vi "BT Tx Test Get Default USL.vi"(8 "error in (no error)":errorcluster, 11 "Template Tx Test in":refnum<class "niDTS BT Tx Test.lvclass">) -> (0 "error out":errorcluster, 2 "Default USL":T1 {"OBW Resutls"."Stop Frequency (Hz)" format="%#_4p"; "OBW Resutls"."Start Frequency (Hz)" format="%#_4p"}, 3 "Template Tx Test out":refnum<class "niDTS BT Tx Test.lvclass">)   [LabVIEW 2015, in "niDTS BT.lvlib" / "niDTS BT Tx Test.lvclass"]
uses:
  niDTS BT Tx Test.lvclass
  Includes/niDTS BT Tx Test INC Results.ctl
  Includes/niDTS BT Tx Test INC IBE Results.ctl
  Includes/niDTS BT Tx Test INC OBW Results.ctl
  Includes/niDTS BT Tx Test INC TXP Results.ctl
  Includes/niDTS BT Tx Test INC DEVM Results.ctl
  Includes/niDTS BT Tx Test INC CF Stability Results.ctl
  Includes/niDTS BT Tx Test INC CFO Resutls.ctl
  Includes/niDTS BT Tx Test INC Character Results.ctl
  niDTS BT Tx Test.lvclass/niDTS BT Tx Test.ctl
  Includes/niDTS BT Tx Test INC Default Limits.vi
  niDTS BT.lvlib
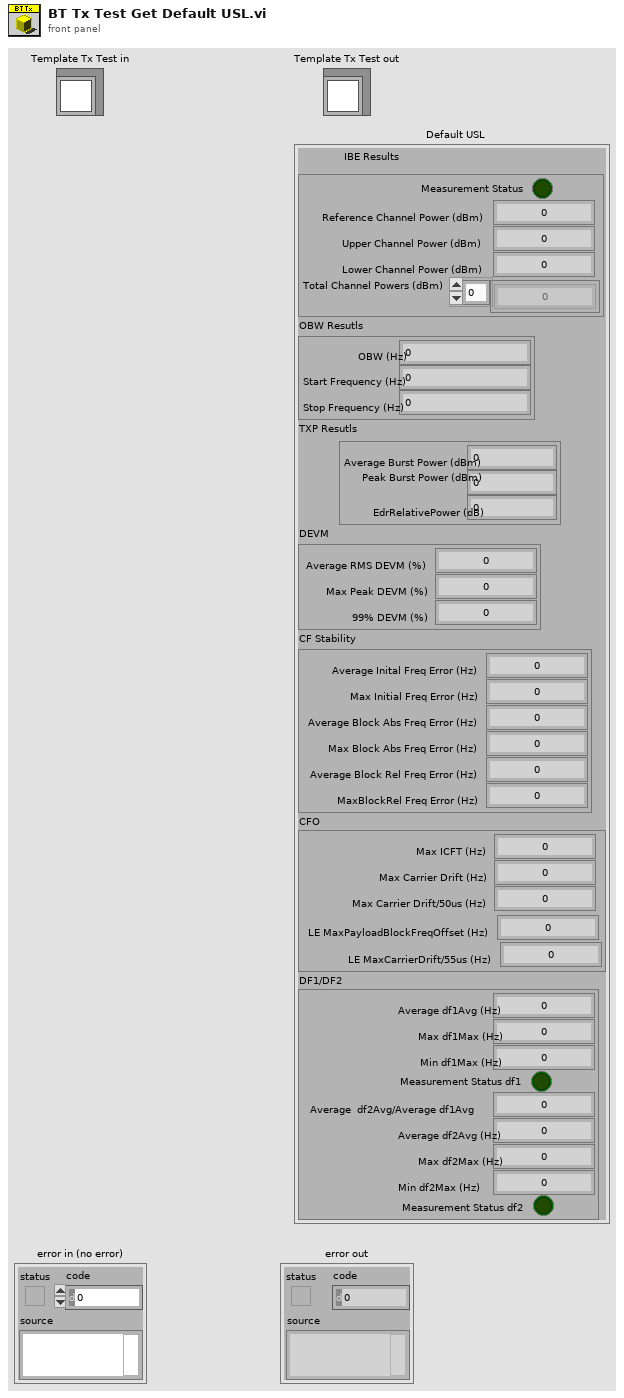
[diagram p1: front panel]
types:
  T1 = typedef "niDTS BT.lvlib/niDTS BT Tx Test INC Results.ctl" = cluster{"IBE Results":T2, "OBW Resutls":T3, "TXP Resutls":T4, "DEVM":T5, "CF Stability":T6, "CFO":T7, "DF1/DF2":T8}
  T2 = typedef "niDTS BT.lvlib/niDTS BT Tx Test INC IBE Results.ctl" = cluster{"Measurement Status":bool, "Reference Channel Power (dBm)":dbl, "Upper Channel Power (dBm)":dbl, "Lower Channel Power (dBm)":dbl, "Total Channel Powers (dBm)":dbl[]}
  T3 = typedef "niDTS BT.lvlib/niDTS BT Tx Test INC OBW Results.ctl" = cluster{"OBW (Hz)":dbl, "Start Frequency (Hz)":dbl, "Stop Frequency (Hz)":dbl}
  T4 = typedef "niDTS BT.lvlib/niDTS BT Tx Test INC TXP Results.ctl" = cluster{"Average Burst Power (dBm)":dbl, "Peak Burst Power (dBm)":dbl, "EdrRelativePower (dB)":dbl}
  T5 = typedef "niDTS BT.lvlib/niDTS BT Tx Test INC DEVM Results.ctl" = cluster{"Average RMS DEVM (%)":dbl, "Max Peak DEVM (%)":dbl, "99% DEVM (%)":dbl}
  T6 = typedef "niDTS BT.lvlib/niDTS BT Tx Test INC CF Stability Results.ctl" = cluster{"Average Inital Freq Error (Hz)":dbl, "Max Initial Freq Error (Hz)":dbl, "Average Block Abs Freq Error (Hz)":dbl, "Max Block Abs Freq Error (Hz)":dbl, "Average Block Rel Freq Error (Hz)":dbl, "MaxBlockRel Freq Error (Hz)":dbl}
  T7 = typedef "niDTS BT.lvlib/niDTS BT Tx Test INC CFO Resutls.ctl" = cluster{"Max ICFT (Hz)":dbl, "Max Carrier Drift (Hz)":dbl, "Max Carrier Drift/50us (Hz)":dbl, "LE MaxPayloadBlockFreqOffset (Hz)":dbl, "LE MaxCarrierDrift/55us (Hz)":dbl}
  T8 = typedef "niDTS BT.lvlib/niDTS BT Tx Test INC Character Results.ctl" = cluster{"Average df1Avg (Hz)":dbl, "Max df1Max (Hz)":dbl, "Min df1Max (Hz)":dbl, "Measurement Status df1":bool, "Average  df2Avg/Average df1Avg":dbl, "Average df2Avg (Hz)":dbl, "Max df2Max (Hz)":dbl, "Min df2Max (Hz)":dbl, "Measurement Status df2":bool}
  T9 = typedef "niDTS BT.lvlib/niDTS BT INC Packet Type.ctl" = enum16{"NULL", "POLL", "FHS", "DM1", "DH1", "HV1", "HV2", "HV3", "EV3", "DV", "AUX1", "DM3", "DH3", "EV4", "EV5", "DM5", "DH5", "LE-TP"}
  T10 = typedef "niDTS BT.lvlib/niDTS BT INC Standard.ctl" = enum16{"BDR", "EDR", "LE-TP"}
  T11 = typedef "niDTS BT.lvlib/niDTS BT Tx Test INC BD Payload Data.ctl" = enum16{"0", "1", "01", "00001111", "PN9", "AUTO"}
  T12 = typedef "niDTS BT.lvlib/niDTS BT Tx Test INC Modulation Characteristics.ctl" = enum16{"DF1", "DF2", "BOTH"}
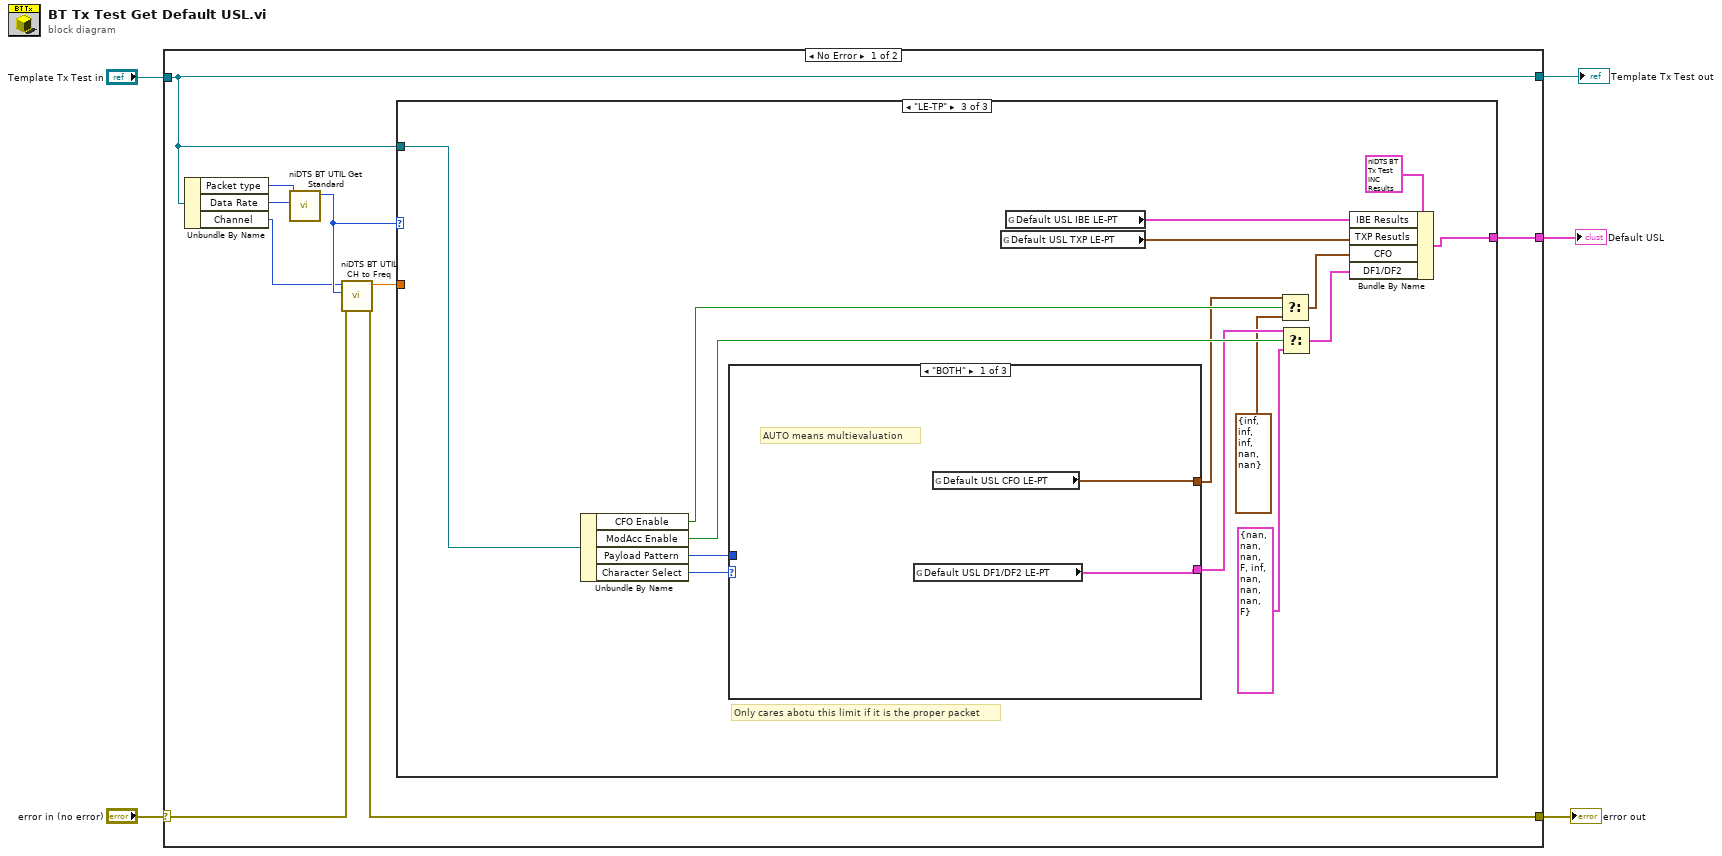
[diagram p0: block diagram]
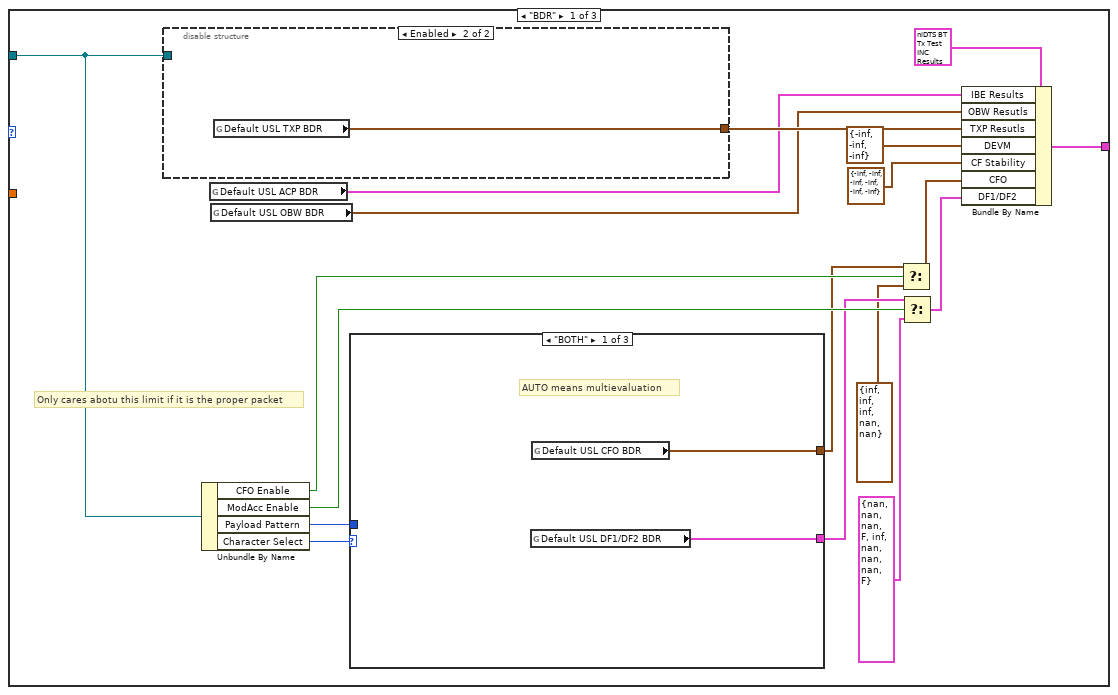
[diagram p2: hidden frame]
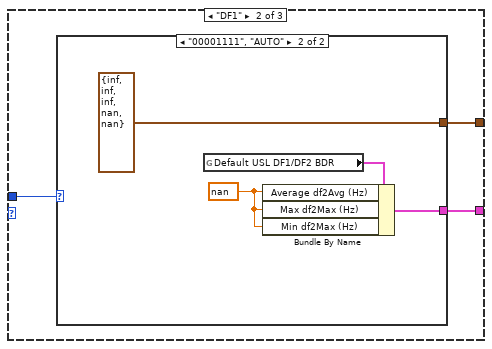
[diagram p3: hidden frame]
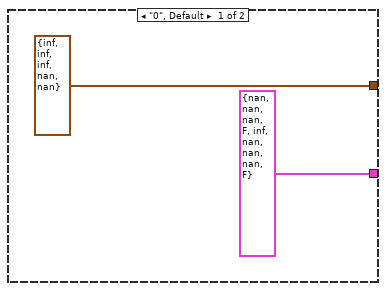
[diagram p4: hidden frame]
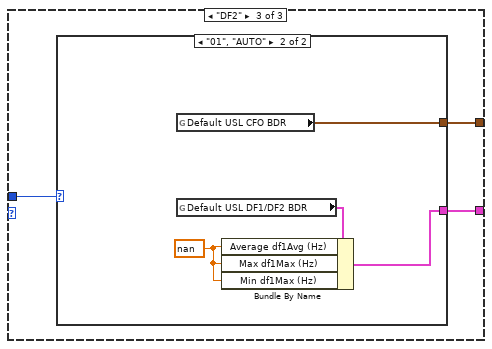
[diagram p5: hidden frame]
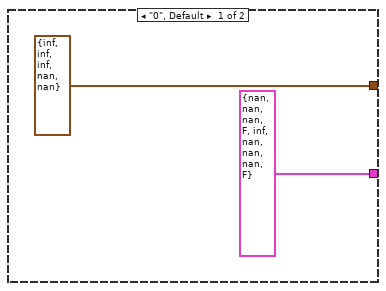
[diagram p6: hidden frame]
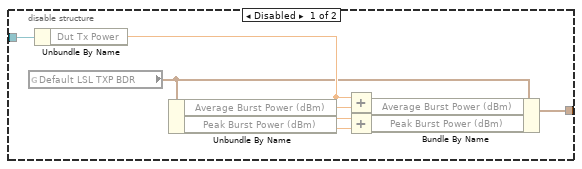
[diagram p7: hidden frame]
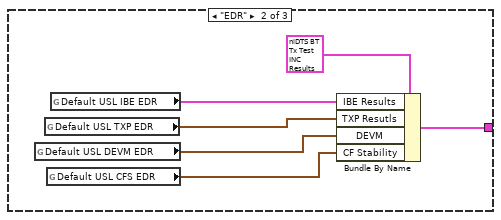
[diagram p8: hidden frame]
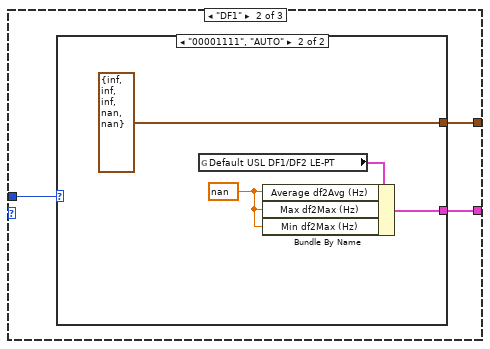
[diagram p9: hidden frame]
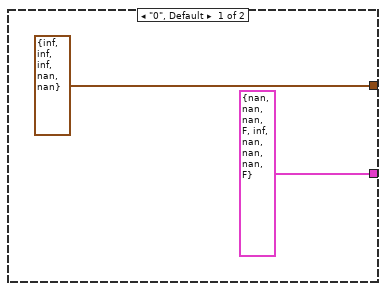
[diagram p10: hidden frame]
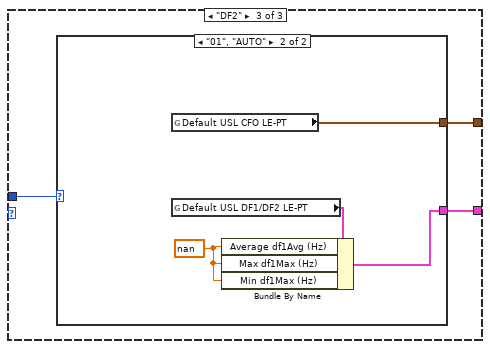
[diagram p11: hidden frame]
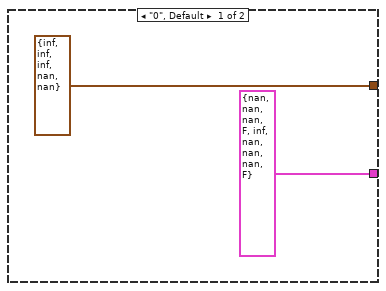
[diagram p12: hidden frame]
diagram:
  n1 = case shown="No Error" "error in (no error)" {
    selector: "error in (no error)" -> [w8 w104]
    tunnel: [w7 w104] -> w1
    tunnel: [w13 w103] -> w3
    tunnel: "Template Tx Test in" -> [w13 w103]
    tunnel: [w14 _] -> w2
    frame No Error {
      n2 = Unbundle By Name(w13) -> ("Packet type"=w11:T9, "Data Rate"=w12:i32, "Channel"=w9:i32)
      n3 = call "niDTS BT UTIL Get Standard.vi"("Data Rate"=w12, "Packet type"=w11) -> ("BT Standard"=w10:T10)  [unwired: 9 in]
      n4 = call "niDTS BT UTIL CH to Freq.vi"("error in (no error)"=w8, "BT Standard"=w10, "Channel"=w9) -> ("error out"=w7:errorcluster, "Frequency"=w6:dbl)  [unwired: 7 in]
      n5 = case shown="\"LE-TP\"" w10 {
        tunnel: [w30 w62 w80] -> w14
        tunnel: w13 -> [w25 _ w71]
        tunnel: w6 -> [_ _ _]
        frame "BDR" {
          # "Only cares abotu this limit if it is the proper packet"
          n6 = disable-structure shown="Enabled" {
            disable-tunnel: w25 -> [w60 _]
            disable-tunnel: [w54 w61] -> w31
            frame Disabled {
              n7 = global read "niDTS BT Tx Test INC Default Limits.vi" "Default LSL TXP BDR"() -> (w53:T4)
              n8 = Unbundle By Name(w60) -> ("Dut Tx Power"=w58:dbl)
              n9 = Unbundle By Name(w53) -> ("Average Burst Power (dBm)"=w59:dbl, "Peak Burst Power (dBm)"=w57:dbl)
              n10 = Add(x=w58, y=w59) -> (x+y=w56:dbl)
              n11 = Add(x=w58, y=w57) -> (x+y=w55:dbl)
              n12 = Bundle By Name(cluster=w53, "Average Burst Power (dBm)"=w56, "Peak Burst Power (dBm)"=w55) -> (w54:T4)
            }
            frame Enabled {
              n13 = global read "niDTS BT Tx Test INC Default Limits.vi" "Default USL TXP BDR"() -> (w61:T4)
            }
          }
          n14 = Unbundle By Name(w25) -> ("CFO Enable"=w23:bool, "ModAcc Enable"=w22:bool, "Payload Pattern"=w24:T11, "Character Select"=w15:T12)
          n15 = global read "niDTS BT Tx Test INC Default Limits.vi" "Default USL ACP BDR"() -> (w29:T2)
          n16 = global read "niDTS BT Tx Test INC Default Limits.vi" "Default USL OBW BDR"() -> (w26:T3)
          n17 = case shown="\"BOTH\"" w15 {
            tunnel: [w33 w37 w46] -> w19
            tunnel: w24 -> [_ w36 w45]
            tunnel: [w34 w35 w44] -> w21
            frame "BOTH" {
              # "AUTO means multievaluation"
              n18 = global read "niDTS BT Tx Test INC Default Limits.vi" "Default USL DF1/DF2 BDR"() -> (w33:T8)
              n19 = global read "niDTS BT Tx Test INC Default Limits.vi" "Default USL CFO BDR"() -> (w34:T7)
            }
            frame "DF1" {
              n20 = case shown="\"00001111\", \"AUTO\"" w36 {
                tunnel: [T8 {"Average df1Avg (Hz)"=nan, "Max df1Max (Hz)"=nan, "Min df1Max (Hz)"=nan, "Measurement Status df1"=FALSE, "Average  df2Avg/Average df1Avg"=inf, "Average df2Avg (Hz)"=nan, "Max df2Max (Hz)"=nan, "Min df2Max (Hz)"=nan, "Measurement Status df2"=FALSE} ("Default USL DF1/DF2 BDR") w41] -> w37
                tunnel: [T7 {"Max ICFT (Hz)"=inf, "Max Carrier Drift (Hz)"=inf, "Max Carrier Drift/50us (Hz)"=inf, "LE MaxPayloadBlockFreqOffset (Hz)"=nan, "LE MaxCarrierDrift/55us (Hz)"=nan} ("f") T7 {"Max ICFT (Hz)"=inf, "Max Carrier Drift (Hz)"=inf, "Max Carrier Drift/50us (Hz)"=inf, "LE MaxPayloadBlockFreqOffset (Hz)"=nan, "LE MaxCarrierDrift/55us (Hz)"=nan} ("f")] -> w35
                frame "0", Default {
                }
                frame "00001111", "AUTO" {
                  w42 = nan ("Average df1Avg")
                  n21 = global read "niDTS BT Tx Test INC Default Limits.vi" "Default USL DF1/DF2 BDR"() -> (w43:T8)
                  n22 = Bundle By Name(cluster=w43, "Average df2Avg (Hz)"=w42, "Max df2Max (Hz)"=w42, "Min df2Max (Hz)"=w42) -> (w41:T8)
                }
              }
            }
            frame "DF2" {
              n23 = case shown="\"01\", \"AUTO\"" w45 {
                tunnel: [T8 {"Average df1Avg (Hz)"=nan, "Max df1Max (Hz)"=nan, "Min df1Max (Hz)"=nan, "Measurement Status df1"=FALSE, "Average  df2Avg/Average df1Avg"=inf, "Average df2Avg (Hz)"=nan, "Max df2Max (Hz)"=nan, "Min df2Max (Hz)"=nan, "Measurement Status df2"=FALSE} ("Default USL DF1/DF2 BDR") w50] -> w46
                tunnel: [T7 {"Max ICFT (Hz)"=inf, "Max Carrier Drift (Hz)"=inf, "Max Carrier Drift/50us (Hz)"=inf, "LE MaxPayloadBlockFreqOffset (Hz)"=nan, "LE MaxCarrierDrift/55us (Hz)"=nan} ("f") w49] -> w44
                frame "0", Default {
                }
                frame "01", "AUTO" {
                  w51 = nan ("Average df1Avg")
                  n24 = global read "niDTS BT Tx Test INC Default Limits.vi" "Default USL CFO BDR"() -> (w49:T7)
                  n25 = global read "niDTS BT Tx Test INC Default Limits.vi" "Default USL DF1/DF2 BDR"() -> (w52:T8)
                  n26 = Bundle By Name(cluster=w52, "Average df1Avg (Hz)"=w51, "Max df1Max (Hz)"=w51, "Min df1Max (Hz)"=w51) -> (w50:T8)
                }
              }
            }
          }
          n27 = Select(t=w21, s=w23, f=T7 {"Max ICFT (Hz)"=inf, "Max Carrier Drift (Hz)"=inf, "Max Carrier Drift/50us (Hz)"=inf, "LE MaxPayloadBlockFreqOffset (Hz)"=nan, "LE MaxCarrierDrift/55us (Hz)"=nan}) -> (s? t:f=w20:T7)
          n28 = Select(t=w19, s=w22, f=T8 {"Average df1Avg (Hz)"=nan, "Max df1Max (Hz)"=nan, "Min df1Max (Hz)"=nan, "Measurement Status df1"=FALSE, "Average  df2Avg/Average df1Avg"=inf, "Average df2Avg (Hz)"=nan, "Max df2Max (Hz)"=nan, "Min df2Max (Hz)"=nan, "Measurement Status df2"=FALSE} ("Default USL DF1/DF2 BDR")) -> (s? t:f=w18:T8)
          n29 = Bundle By Name(cluster=T1 {"IBE Results"={"Measurement Status"=FALSE, "Reference Channel Power (dBm)"=0.0, "Upper Channel Power (dBm)"=0.0, "Lower Channel Power (dBm)"=0.0, "Total Channel Powers (dBm)"=[]}, "OBW Resutls"={"OBW (Hz)"=0.0, "Start Frequency (Hz)"=0.0, "Stop Frequency (Hz)"=0.0}, "TXP Resutls"={"Average Burst Power (dBm)"=-35.0, "Peak Burst Power (dBm)"=-35.0, "EdrRelativePower (dB)"=0.0}, "DEVM"={"Average RMS DEVM (%)"=0.0, "Max Peak DEVM (%)"=0.0, "99% DEVM (%)"=0.0}, "CF Stability"={"Average Inital Freq Error (Hz)"=0.0, "Max Initial Freq Error (Hz)"=0.0, "Average Block Abs Freq Error (Hz)"=0.0, "Max Block Abs Freq Error (Hz)"=0.0, "Average Block Rel Freq Error (Hz)"=0.0, "MaxBlockRel Freq Error (Hz)"=0.0}, "CFO"={"Max ICFT (Hz)"=0.0, "Max Carrier Drift (Hz)"=0.0, "Max Carrier Drift/50us (Hz)"=0.0, "LE MaxPayloadBlockFreqOffset (Hz)"=0.0, "LE MaxCarrierDrift/55us (Hz)"=0.0}, "DF1/DF2"={"Average df1Avg (Hz)"=0.0, "Max df1Max (Hz)"=0.0, "Min df1Max (Hz)"=0.0, "Measurement Status df1"=FALSE, "Average  df2Avg/Average df1Avg"=0.0, "Average df2Avg (Hz)"=0.0, "Max df2Max (Hz)"=0.0, "Min df2Max (Hz)"=0.0, "Measurement Status df2"=FALSE}} ("Default USL"), "IBE Results"=w29, "OBW Resutls"=w26, "TXP Resutls"=w31, "DEVM"=T5 {"Average RMS DEVM (%)"=-inf, "Max Peak DEVM (%)"=-inf, "99% DEVM (%)"=-inf}, "CF Stability"=T6 {"Average Inital Freq Error (Hz)"=-inf, "Max Initial Freq Error (Hz)"=-inf, "Average Block Abs Freq Error (Hz)"=-inf, "Max Block Abs Freq Error (Hz)"=-inf, "Average Block Rel Freq Error (Hz)"=-inf, "MaxBlockRel Freq Error (Hz)"=-inf}, "CFO"=w20, "DF1/DF2"=w18) -> (w30:T1)
        }
        frame "EDR" {
          n30 = global read "niDTS BT Tx Test INC Default Limits.vi" "Default USL DEVM EDR"() -> (w64:T5)
          n31 = global read "niDTS BT Tx Test INC Default Limits.vi" "Default USL TXP EDR"() -> (w63:T4)
          n32 = global read "niDTS BT Tx Test INC Default Limits.vi" "Default USL CFS EDR"() -> (w65:T6)
          n33 = global read "niDTS BT Tx Test INC Default Limits.vi" "Default USL IBE EDR"() -> (w66:T2)
          n34 = Bundle By Name(cluster=T1 {"IBE Results"={"Measurement Status"=FALSE, "Reference Channel Power (dBm)"=0.0, "Upper Channel Power (dBm)"=0.0, "Lower Channel Power (dBm)"=0.0, "Total Channel Powers (dBm)"=[]}, "OBW Resutls"={"OBW (Hz)"=0.0, "Start Frequency (Hz)"=0.0, "Stop Frequency (Hz)"=0.0}, "TXP Resutls"={"Average Burst Power (dBm)"=-35.0, "Peak Burst Power (dBm)"=-35.0, "EdrRelativePower (dB)"=0.0}, "DEVM"={"Average RMS DEVM (%)"=0.0, "Max Peak DEVM (%)"=0.0, "99% DEVM (%)"=0.0}, "CF Stability"={"Average Inital Freq Error (Hz)"=0.0, "Max Initial Freq Error (Hz)"=0.0, "Average Block Abs Freq Error (Hz)"=0.0, "Max Block Abs Freq Error (Hz)"=0.0, "Average Block Rel Freq Error (Hz)"=0.0, "MaxBlockRel Freq Error (Hz)"=0.0}, "CFO"={"Max ICFT (Hz)"=0.0, "Max Carrier Drift (Hz)"=0.0, "Max Carrier Drift/50us (Hz)"=0.0, "LE MaxPayloadBlockFreqOffset (Hz)"=0.0, "LE MaxCarrierDrift/55us (Hz)"=0.0}, "DF1/DF2"={"Average df1Avg (Hz)"=0.0, "Max df1Max (Hz)"=0.0, "Min df1Max (Hz)"=0.0, "Measurement Status df1"=FALSE, "Average  df2Avg/Average df1Avg"=0.0, "Average df2Avg (Hz)"=0.0, "Max df2Max (Hz)"=0.0, "Min df2Max (Hz)"=0.0, "Measurement Status df2"=FALSE}} ("Default USL"), "IBE Results"=w66, "TXP Resutls"=w63, "DEVM"=w64, "CF Stability"=w65) -> (w62:T1)
        }
        frame "LE-TP" {
          # "Only cares abotu this limit if it is the proper packet"
          n35 = Unbundle By Name(w71) -> ("CFO Enable"=w78:bool, "ModAcc Enable"=w77:bool, "Payload Pattern"=w79:T11, "Character Select"=w72:T12)
          n36 = case shown="\"BOTH\"" w72 {
            tunnel: [w83 w87 w96] -> w75
            tunnel: w79 -> [_ w86 w95]
            tunnel: [w84 w85 w94] -> w76
            frame "BOTH" {
              # "AUTO means multievaluation"
              n37 = global read "niDTS BT Tx Test INC Default Limits.vi" "Default USL DF1/DF2 LE-PT"() -> (w83:T8)
              n38 = global read "niDTS BT Tx Test INC Default Limits.vi" "Default USL CFO LE-PT"() -> (w84:T7)
            }
            frame "DF1" {
              n39 = case shown="\"00001111\", \"AUTO\"" w86 {
                tunnel: [T8 {"Average df1Avg (Hz)"=nan, "Max df1Max (Hz)"=nan, "Min df1Max (Hz)"=nan, "Measurement Status df1"=FALSE, "Average  df2Avg/Average df1Avg"=inf, "Average df2Avg (Hz)"=nan, "Max df2Max (Hz)"=nan, "Min df2Max (Hz)"=nan, "Measurement Status df2"=FALSE} ("Default USL DF1/DF2 BDR") w91] -> w87
                tunnel: [T7 {"Max ICFT (Hz)"=inf, "Max Carrier Drift (Hz)"=inf, "Max Carrier Drift/50us (Hz)"=inf, "LE MaxPayloadBlockFreqOffset (Hz)"=nan, "LE MaxCarrierDrift/55us (Hz)"=nan} ("f") T7 {"Max ICFT (Hz)"=inf, "Max Carrier Drift (Hz)"=inf, "Max Carrier Drift/50us (Hz)"=inf, "LE MaxPayloadBlockFreqOffset (Hz)"=nan, "LE MaxCarrierDrift/55us (Hz)"=nan} ("f")] -> w85
                frame "0", Default {
                }
                frame "00001111", "AUTO" {
                  w92 = nan ("Average df1Avg")
                  n40 = global read "niDTS BT Tx Test INC Default Limits.vi" "Default USL DF1/DF2 LE-PT"() -> (w93:T8)
                  n41 = Bundle By Name(cluster=w93, "Average df2Avg (Hz)"=w92, "Max df2Max (Hz)"=w92, "Min df2Max (Hz)"=w92) -> (w91:T8)
                }
              }
            }
            frame "DF2" {
              n42 = case shown="\"01\", \"AUTO\"" w95 {
                tunnel: [T8 {"Average df1Avg (Hz)"=nan, "Max df1Max (Hz)"=nan, "Min df1Max (Hz)"=nan, "Measurement Status df1"=FALSE, "Average  df2Avg/Average df1Avg"=inf, "Average df2Avg (Hz)"=nan, "Max df2Max (Hz)"=nan, "Min df2Max (Hz)"=nan, "Measurement Status df2"=FALSE} ("Default USL DF1/DF2 BDR") w100] -> w96
                tunnel: [T7 {"Max ICFT (Hz)"=inf, "Max Carrier Drift (Hz)"=inf, "Max Carrier Drift/50us (Hz)"=inf, "LE MaxPayloadBlockFreqOffset (Hz)"=nan, "LE MaxCarrierDrift/55us (Hz)"=nan} ("f") w99] -> w94
                frame "0", Default {
                }
                frame "01", "AUTO" {
                  w101 = nan ("Average df1Avg")
                  n43 = global read "niDTS BT Tx Test INC Default Limits.vi" "Default USL CFO LE-PT"() -> (w99:T7)
                  n44 = global read "niDTS BT Tx Test INC Default Limits.vi" "Default USL DF1/DF2 LE-PT"() -> (w102:T8)
                  n45 = Bundle By Name(cluster=w102, "Average df1Avg (Hz)"=w101, "Max df1Max (Hz)"=w101, "Min df1Max (Hz)"=w101) -> (w100:T8)
                }
              }
            }
          }
          n46 = global read "niDTS BT Tx Test INC Default Limits.vi" "Default USL TXP LE-PT"() -> (w70:T4)
          n47 = global read "niDTS BT Tx Test INC Default Limits.vi" "Default USL IBE LE-PT"() -> (w81:T2)
          n48 = Select(t=w76, s=w78, f=T7 {"Max ICFT (Hz)"=inf, "Max Carrier Drift (Hz)"=inf, "Max Carrier Drift/50us (Hz)"=inf, "LE MaxPayloadBlockFreqOffset (Hz)"=nan, "LE MaxCarrierDrift/55us (Hz)"=nan}) -> (s? t:f=w69:T7)
          n49 = Select(t=w75, s=w77, f=T8 {"Average df1Avg (Hz)"=nan, "Max df1Max (Hz)"=nan, "Min df1Max (Hz)"=nan, "Measurement Status df1"=FALSE, "Average  df2Avg/Average df1Avg"=inf, "Average df2Avg (Hz)"=nan, "Max df2Max (Hz)"=nan, "Min df2Max (Hz)"=nan, "Measurement Status df2"=FALSE} ("Default USL DF1/DF2 BDR")) -> (s? t:f=w68:T8)
          n50 = Bundle By Name(cluster=T1 {"IBE Results"={"Measurement Status"=FALSE, "Reference Channel Power (dBm)"=0.0, "Upper Channel Power (dBm)"=0.0, "Lower Channel Power (dBm)"=0.0, "Total Channel Powers (dBm)"=[]}, "OBW Resutls"={"OBW (Hz)"=0.0, "Start Frequency (Hz)"=0.0, "Stop Frequency (Hz)"=0.0}, "TXP Resutls"={"Average Burst Power (dBm)"=-35.0, "Peak Burst Power (dBm)"=-35.0, "EdrRelativePower (dB)"=0.0}, "DEVM"={"Average RMS DEVM (%)"=0.0, "Max Peak DEVM (%)"=0.0, "99% DEVM (%)"=0.0}, "CF Stability"={"Average Inital Freq Error (Hz)"=0.0, "Max Initial Freq Error (Hz)"=0.0, "Average Block Abs Freq Error (Hz)"=0.0, "Max Block Abs Freq Error (Hz)"=0.0, "Average Block Rel Freq Error (Hz)"=0.0, "MaxBlockRel Freq Error (Hz)"=0.0}, "CFO"={"Max ICFT (Hz)"=0.0, "Max Carrier Drift (Hz)"=0.0, "Max Carrier Drift/50us (Hz)"=0.0, "LE MaxPayloadBlockFreqOffset (Hz)"=0.0, "LE MaxCarrierDrift/55us (Hz)"=0.0}, "DF1/DF2"={"Average df1Avg (Hz)"=0.0, "Max df1Max (Hz)"=0.0, "Min df1Max (Hz)"=0.0, "Measurement Status df1"=FALSE, "Average  df2Avg/Average df1Avg"=0.0, "Average df2Avg (Hz)"=0.0, "Max df2Max (Hz)"=0.0, "Min df2Max (Hz)"=0.0, "Measurement Status df2"=FALSE}} ("Default USL"), "IBE Results"=w81, "TXP Resutls"=w70, "CFO"=w69, "DF1/DF2"=w68) -> (w80:T1)
        }
      }
    }
    frame Error {
    }
  }
  "error out" <- w1
  "Template Tx Test out" <- w3
  "Default USL" <- w2
